vi "uev_create_user_event_stop.vi"(8 "error in (no error)":errorcluster) -> (0 "error out":errorcluster, 2 "User Event - Stop":refnum<user-event>, 3 "Stop Event Registration Refnum":refnum<event-registration>)   [LabVIEW 2013]
doc: "Create a boolean user event that will be used to stop the event loop from the message handling loop."
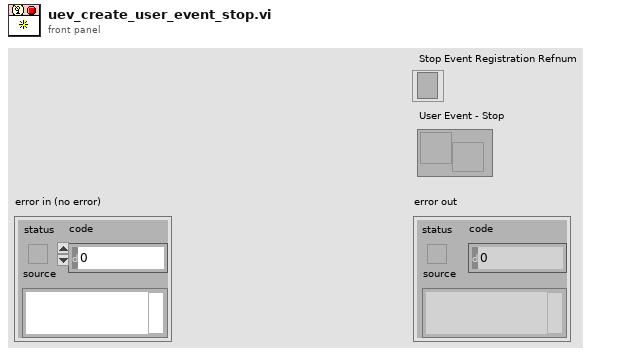
[diagram p1: front panel]
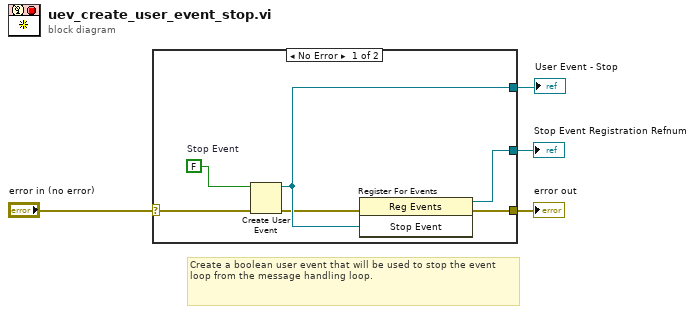
[diagram p0: block diagram]
diagram:
  # "Create a boolean user event that will be used to stop the event loop from the message handling loop."
  n1 = case shown="No Error" "error in (no error)" {
    selector: "error in (no error)" -> [w6 w11]
    tunnel: [w10 _] -> w2
    tunnel: [w9 _] -> w1
    tunnel: [w7 w11] -> w4
    frame No Error {
      w5 = FALSE  # Stop Event
      n2 = Create User Event(user event datatype=w5, error in=w6) -> (user event=w10:refnum<user-event>, error out=w8:errorcluster)
      n3 = register-events(error in=w8, w10) -> (reference out=w9:refnum<event-registration>, error out=w7:errorcluster)  [unwired: 1 in]
    }
    frame Error {
    }
  }
  "User Event - Stop" <- w2
  "error out" <- w4
  "Stop Event Registration Refnum" <- w1
